vi "ControlValueToJSON.vi"(7 "UseEnum":bool=TRUE, 8 "error in (no error)":errorcluster, 10 "Value":variant, 11 "Control in":refnum<vi>) -> (0 "error out":errorcluster, 3 "String":string)   [LabVIEW 2019]
uses:
  <vilib>/Utility/Data Type/NI_Data Type.lvlib
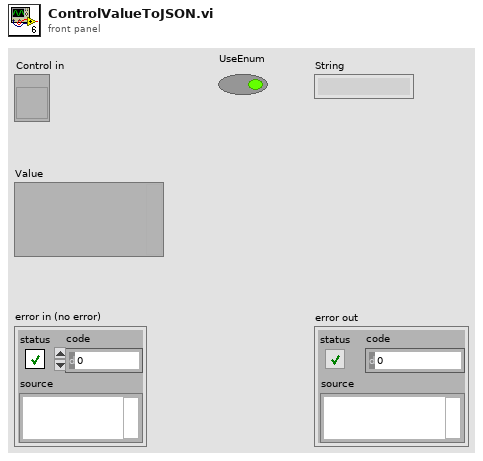
[diagram p1: front panel]
types:
  T1 = typedef "NI_Data Type.lvlib/Data Type.ctl" = enum8{"Invalid Type", "Void", "I8", "I16", "I32", "I64", "U8", "U16", "U32", "U64", "Single Float", "Double Float", "Extended Float", "Single Complex", "Double Complex", "Extended Complex", "Enum U8", "Enum U16", "Enum U32", "Enum U64", "Single Float With Unit", "Double Float With Unit", "Extended Float With Unit", "Single Complex with Unit", "Double Complex with Unit", "Extended Complex with Unit", "Boolean", "String", "Path", "Picture", "Tag", "Array", "Cluster", "Variant", "LV Variant", "Waveform", "Timestamp", "Digital Waveform", "Digital Data", "ExpressData", "Refnum", "External Data", "VI", "Poly VI", "LabVIEW Class Instance", "Fixed Point", "Set Collection", "Map Collection"}
  T2 = typedef "LVStringsAndValuesArrayTypeDef.ctl" = cluster{"String":string, "Value":ext}[]
  T3 = typedef "NI_Data Type.lvlib/Refnum Type.ctl" = enum16{"NotARefnum", "UnknownRefnum", "Generic", "Datalog", "ByteStream", "Device", "Occurence", "TCPNetConnection", "Auto", "Menu", "Imaq", "Hardware", "DataSocket", "Visa", "IVI", "UDPNetConnection", "Notifier", "Queue", "Irda", "EventReg", "DotNet", "UserEvent", "Callback", "UNUSED_EMPTY_POSITION", "BlueToothNetConnection", "LVObjApp", "LVObjVI", "LVObjUnknown", "GenericClass", "UserDefinedRefnumTag", "DataValue", "RT FIFO", "TDMS File", "PythonSessionRefnum"}
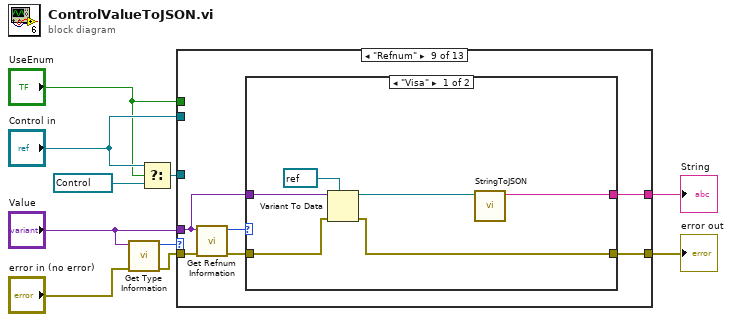
[diagram p0: block diagram]
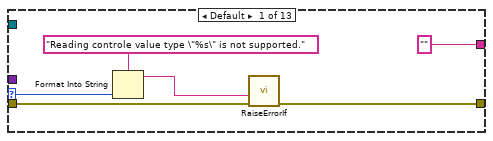
[diagram p2: hidden frame]
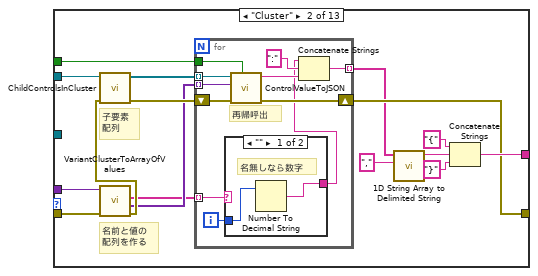
[diagram p3: hidden frame]
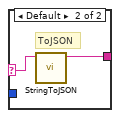
[diagram p4: hidden frame]
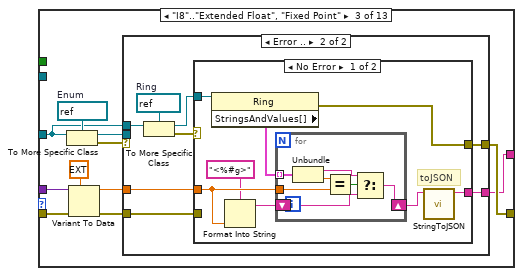
[diagram p5: hidden frame]
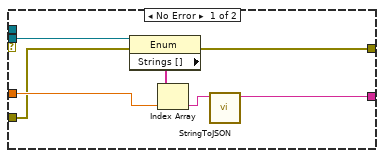
[diagram p6: hidden frame]
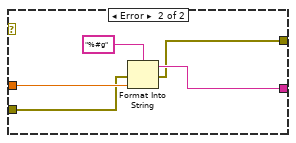
[diagram p7: hidden frame]
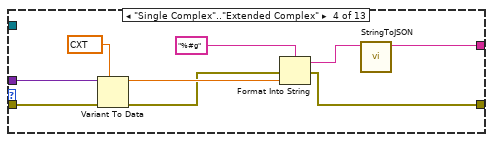
[diagram p8: hidden frame]
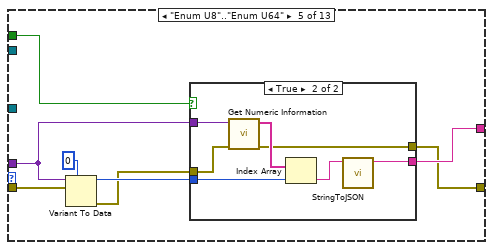
[diagram p9: hidden frame]
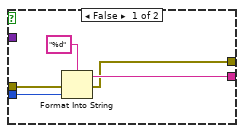
[diagram p10: hidden frame]
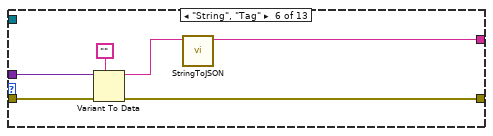
[diagram p11: hidden frame]
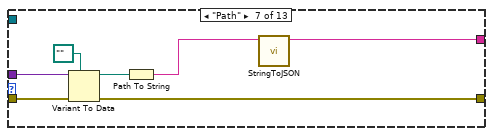
[diagram p12: hidden frame]
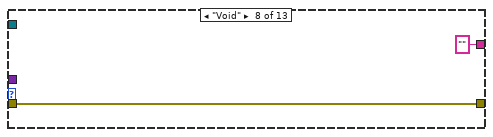
[diagram p13: hidden frame]
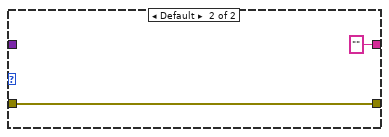
[diagram p14: hidden frame]
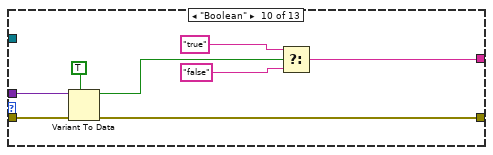
[diagram p15: hidden frame]
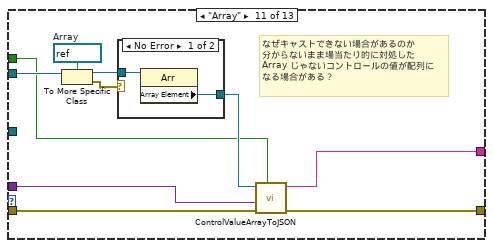
[diagram p16: hidden frame]
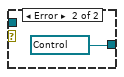
[diagram p17: hidden frame]
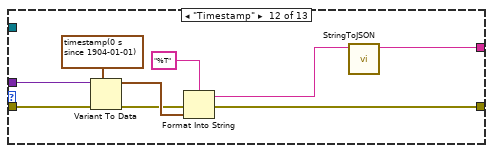
[diagram p18: hidden frame]
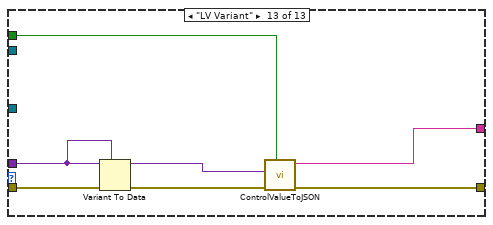
[diagram p19: hidden frame]
diagram:
  n1 = call <vilib>:"Get Type Information.vi"("error in (no error)"="error in (no error)", "variant"="Value") -> ("error out"=w4:errorcluster, "type"=w8:T1)  [unwired: 5 in, 3 out]
  n2 = Select(t="Control in", s="UseEnum", f=refnum<vi> refnum) -> (s? t:f=w7:refnum<vi>)
  n3 = case shown="\"Refnum\"" w8 {
    selector: w8 -> [w14 _ _ _ _ _ _ _ _ _ _ _ _]
    tunnel: ["" ("f") w24 w50 w94 w107 w123 w129 "" ("f") w141 w154 w169 w175 w187] -> w9
    tunnel: "Value" -> [_ w22 w58 w98 w109 w127 w135 _ w142 w159 w161 w181 w183]
    tunnel: w7 -> [_ _ w48 _ _ _ _ _ _ _ _ _ _]
    tunnel: w4 -> [w13 w21 w53 w97 w106 w126 w133 w136 w140 w153 w162 w173 w185]
    tunnel: [w12 w23 w51 w96 w104 w125 w131 w136 w138 w152 w168 w177 w186] -> w3
    tunnel: "Control in" -> [_ w32 _ _ _ _ _ _ _ _ w167 _ _]
    tunnel: "UseEnum" -> [_ w30 _ _ w103 _ _ _ _ _ w160 _ w188]
    frame Default {
      n4 = Format Into String(format string="Reading controle value type \"%s\" is not supported.", w14) -> (resulting string=w11:string)  [unwired: 2 in, 1 out]
      n5 = call "RaiseErrorIf.vi"("error in (no error)"=w13, "error message"=w11) -> ("error out"=w12:errorcluster)  [unwired: 9 in]
    }
    frame "Cluster" {
      # "名前と値の\n配列を作る"
      # "子要素\n配列"
      n6 = call "VariantClusterToArrayOfValues.vi"("error in (no error)"=w21, "Cluster Variant"=w22) -> ("error out"=w20:errorcluster, "Values"=w19:variant[], "Names"=w18:string[])  [unwired: 7 in]
      n7 = call "ChildControlsInCluster.vi"("error in (no error)"=w20, "Control in"=w32) -> ("error out"=w29:errorcluster, "Controls[]"=w31:refnum<vi>[])  [unwired: 7 in, 1 out]
      n8 = for {
        tunnel: w31 -> [w41] mode=indexing
        tunnel: w30 -> [w43]
        shift-right: [w34] -> w23
        shift-left: w29 -> [w42]
        tunnel: [w38] -> w17 mode=indexing
        tunnel: w19 -> [w37] mode=indexing
        tunnel: w18 -> [w35] mode=indexing
        i -> [w36]
        # "再帰呼出"
        n9 = case shown="\"\"" w35 {
          selector: w35 -> [_ w46]
          tunnel: [w44 w47] -> w33
          tunnel: w36 -> [w45 _]
          frame "" {
            # "名無しなら数字"
            n10 = Number To Decimal String(number=w45) -> (decimal integer string=w44:string)  [unwired: 1 in]
          }
          frame Default {
            # "ToJSON"
            n11 = call "StringToJSON.vi"("input text"=w46) -> ("JSON string"=w47:string)  [unwired: 10 in]
          }
        }
        n12 = call "ControlValueToJSON.vi"("UseEnum"=w43, "error in (no error)"=w42, "Value"=w37, "Control in"=w41) -> ("error out"=w34:errorcluster, "String"=w39:string)  [unwired: 6 in]
        n13 = Concatenate Strings(w33, ":" ("string"), w39) -> (w38:string)
      }
      n14 = call <vilib>:"1D String Array to Delimited String.vi"("delimiter"=",", "string array"=w17) -> ("delimited string"=w26:string)  [unwired: 9 in]
      n15 = Concatenate Strings("{" ("string"), w26, "}" ("string")) -> (w24:string)
    }
    frame "I8".."Extended Float", "Fixed Point" {
      w56 = refnum<vi> refnum  # Enum
      n16 = To More Specific Class(target class=w56, reference=w48) -> (specific class reference=w54:refnum<vi>, error out=w55:errorcluster)  [unwired: 1 in]
      n17 = Variant To Data(error in=w53, type=ext 0.0 ("number"), Variant=w58) -> (data=w57:ext, error out=w52:errorcluster)
      n18 = case shown="Error .." w55 {
        tunnel: w57 -> [w63 w73]
        tunnel: [w59 w72] -> w50
        tunnel: w54 -> [w65 _]
        tunnel: w52 -> [w62 w71]
        tunnel: [w61 w70] -> w51
        tunnel: w48 -> [_ w68]
        frame No Error {
          n19 = property class="Enum"(reference=w65, error in=w62) -> (error out=w61:errorcluster, "Strings []"=w64:string[])  [unwired: 1 out]
          n20 = Index Array(array=w64, index=w63) -> (element=w60:string)
          n21 = call "StringToJSON.vi"("input text"=w60) -> ("JSON string"=w59:string)  [unwired: 10 in]
        }
        frame Error {
          w69 = refnum<vi> refnum  # Ring
          n22 = To More Specific Class(target class=w69, reference=w68) -> (specific class reference=w66:refnum<vi>, error out=w67:errorcluster)  [unwired: 1 in]
          n23 = case shown="No Error" w67 {
            tunnel: w73 -> [w76 w92]
            tunnel: [w78 w91] -> w72
            tunnel: w71 -> [_ w90]
            tunnel: [w79 w89] -> w70
            tunnel: w66 -> [w81 _]
            frame No Error {
              # "toJSON"
              n24 = property class="Ring"(reference=w81) -> (error out=w79:errorcluster, "StringsAndValues[]"=w80:T2)  [unwired: 1 in, 1 out]
              n25 = Format Into String(format string="<%#g>", w76) -> (resulting string=w74:string)  [unwired: 2 in, 1 out]
              n26 = for {
                tunnel: w80 -> [w88] mode=indexing
                tunnel: w76 -> [w86]
                shift-right: [w83] -> w77
                shift-left: w74 -> [w82]
                n27 = Unbundle(w88) -> ("String"=w84:string, "Value"=w87:ext)
                n28 = Equal?(x=w87, y=w86) -> (x = y?=w85:bool)
                n29 = Select(t=w84, s=w85, f=w82) -> (s? t:f=w83:string)
              }
              n30 = call "StringToJSON.vi"("input text"=w77) -> ("JSON string"=w78:string)  [unwired: 10 in]
            }
            frame Error {
              n31 = Format Into String(format string="%#g", error in=w90, w92) -> (resulting string=w91:string, error out=w89:errorcluster)  [unwired: 1 in]
            }
          }
        }
      }
    }
    frame "Single Complex".."Extended Complex" {
      n32 = Variant To Data(error in=w97, type=cxt 0.0+0.0i ("number"), Variant=w98) -> (data=w100:cxt, error out=w99:errorcluster)
      n33 = Format Into String(format string="%#g", error in=w99, w100) -> (resulting string=w95:string, error out=w96:errorcluster)  [unwired: 1 in]
      n34 = call "StringToJSON.vi"("input text"=w95) -> ("JSON string"=w94:string)  [unwired: 10 in]
    }
    frame "Enum U8".."Enum U64" {
      n35 = Variant To Data(error in=w106, type=u64 0, Variant=w109) -> (data=w108:u64, error out=w105:errorcluster)
      n36 = case shown="True" w103 {
        tunnel: w109 -> [_ w122]
        tunnel: w108 -> [w114 w120]
        tunnel: [w113 w116] -> w107
        tunnel: w105 -> [w112 w119]
        tunnel: [w111 w118] -> w104
        frame False {
          n37 = Format Into String(format string="%d", error in=w112, w114) -> (resulting string=w113:string, error out=w111:errorcluster)  [unwired: 1 in]
        }
        frame True {
          n38 = call <vilib>:"Get Numeric Information.vi"("error in (no error)"=w119, "variant"=w122) -> ("error out"=w118:errorcluster, "enum names"=w121:string[])  [unwired: 6 in, 2 out]
          n39 = Index Array(array=w121, index=w120) -> (element=w117:string)
          n40 = call "StringToJSON.vi"("input text"=w117) -> ("JSON string"=w116:string)  [unwired: 10 in]
        }
      }
    }
    frame "String", "Tag" {
      n41 = Variant To Data(error in=w126, type="", Variant=w127) -> (data=w124:string, error out=w125:errorcluster)
      n42 = call "StringToJSON.vi"("input text"=w124) -> ("JSON string"=w123:string)  [unwired: 10 in]
    }
    frame "Path" {
      n43 = Variant To Data(error in=w133, type=path "" ("path"), Variant=w135) -> (data=w132:path, error out=w131:errorcluster)
      n44 = Path To String(path=w132) -> (string=w130:string)
      n45 = call "StringToJSON.vi"("input text"=w130) -> ("JSON string"=w129:string)  [unwired: 10 in]
    }
    frame "Void" {
    }
    frame "Refnum" {
      n46 = call <vilib>:"Get Refnum Information.vi"("error in (no error)"=w140, "variant"=w142) -> ("error out"=w139:errorcluster, "reference type"=w143:T3)  [unwired: 6 in, 2 out]
      n47 = case shown="\"Visa\"" w143 {
        tunnel: w142 -> [w148 _]
        tunnel: [w147 "" ("JSON string")] -> w141
        tunnel: w139 -> [w146 w151]
        tunnel: [w144 w151] -> w138
        frame "Visa" {
          n48 = Variant To Data(error in=w146, type=refnum<visa-resource-name> refnum ("VISA resource name out"), Variant=w148) -> (data=w145:refnum<visa-resource-name>, error out=w144:errorcluster)
          n49 = call "StringToJSON.vi"("input text"=w145) -> ("JSON string"=w147:string)  [unwired: 10 in]
        }
        frame Default {
        }
      }
    }
    frame "Boolean" {
      n50 = Variant To Data(error in=w153, type=TRUE, Variant=w159) -> (data=w157:bool, error out=w152:errorcluster)
      n51 = Select(t="true", s=w157, f="false") -> (s? t:f=w154:string)
    }
    frame "Array" {
      w165 = refnum<vi> refnum  # Array
      # "なぜキャストできない場合があるのか\n分からないまま場当たり的に対処した\nArray じゃないコントロールの値が配列に\nなる場合がある？"
      n52 = To More Specific Class(target class=w165, reference=w167) -> (specific class reference=w166:refnum<vi>, error out=w163:errorcluster)  [unwired: 1 in]
      n53 = case shown="No Error" w163 {
        tunnel: w166 -> [w171 _]
        tunnel: [w170 refnum<vi> refnum ("f")] -> w164
        frame No Error {
          n54 = property class="Arr"(reference=w171) -> ("Array Element"=w170:refnum<vi>)  [unwired: 1 in, 2 out]
        }
        frame Error {
        }
      }
      n55 = call "ControlValueArrayToJSON.vi"("UseEnum"=w160, "error in (no error)"=w162, "Array in"=w161, "Control in"=w164) -> ("error out"=w168:errorcluster, "String out"=w169:string)  [unwired: 6 in]
    }
    frame "Timestamp" {
      n56 = Variant To Data(error in=w173, type=timestamp(0 s since 1904-01-01) ("time stamp"), Variant=w181) -> (data=w179:timestamp, error out=w178:errorcluster)
      n57 = Format Into String(format string="%T", error in=w178, w179) -> (resulting string=w176:string, error out=w177:errorcluster)  [unwired: 1 in]
      n58 = call "StringToJSON.vi"("input text"=w176) -> ("JSON string"=w175:string)  [unwired: 10 in]
    }
    frame "LV Variant" {
      n59 = Variant To Data(error in=w185, type=w183, Variant=w183) -> (data=w182:variant, error out=w184:errorcluster)
      n60 = call "ControlValueToJSON.vi"("UseEnum"=w188, "error in (no error)"=w184, "Value"=w182) -> ("error out"=w186:errorcluster, "String"=w187:string)  [unwired: 7 in]
    }
  }
  "String" <- w9
  "error out" <- w3
